vi "Mask Errors.vi"(7 "Severity":T1=enum."Warning", 8 "Error In":errorcluster, 11 "Error Codes":i32[](array[numeric])) -> (0 "Error Out":errorcluster, 3 "Found?":bool)   [LabVIEW 2017, in "Toolkit.lvlib"]
doc: "Masks and clears any error that matches the error codes listed. Masking changes an error from Recoverable or Fatal to either a Warning or Benign."
uses:
  Toolkit.lvlib
  Controls/Severity.ctl
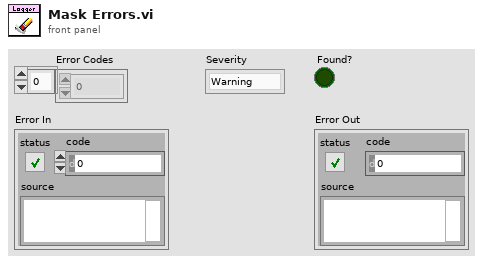
[diagram p1: front panel]
types:
  T1 = typedef "Toolkit.lvlib/Severity.ctl" = enum16{"Benign", "Warning", "Recoverable", "Fatal"}
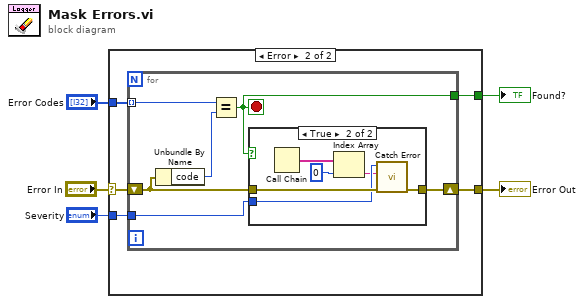
[diagram p0: block diagram]
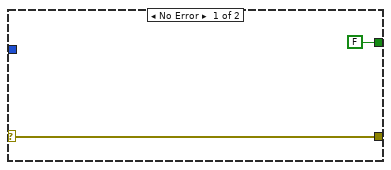
[diagram p2: hidden frame]
diagram:
  n1 = case shown="Error" "Error In" {
    selector: "Error In" -> [w7 w12]
    tunnel: "Error Codes" -> [_ w11]
    tunnel: [w7 w10] -> w3
    tunnel: [FALSE w9] -> w2
    tunnel: "Severity" -> [_ w8]
    frame No Error {
    }
    frame Error {
      n2 = for {
        shift-right: [w15] -> w10
        shift-left: w12 -> [w16]
        tunnel: w11 -> [w17] mode=indexing
        tunnel: [w14] -> w9
        tunnel: w8 -> [w13]
        stop <- w14 stop-if-true
        n3 = Unbundle By Name(w16) -> ("code"=w18:i32)
        n4 = Equal?(x=w17, y=w18) -> (x = y?=w14:bool)
        n5 = case shown="True" w14 {
          tunnel: w16 -> [w19 w25]
          tunnel: [w19 w24] -> w15
          tunnel: w13 -> [_ w23]
          frame False {
          }
          frame True {
            n6 = Call Chain() -> (call chain=w22:string[])
            n7 = Index Array(array=w22, index=0) -> (element=w20:string)
            n8 = call "Catch Error.vi"("Error In"=w25, "Source"=w20, "Severity"=w23) -> ("Error Out"=w24:errorcluster)  [unwired: 8 in]
          }
        }
      }
    }
  }
  "Error Out" <- w3
  "Found?" <- w2
